vi "Get Category.vi"(8 "error in (no error)":errorcluster, 11 "WaveformAcq editor node in":refnum<class "WaveformAcq editor node.lvclass">) -> (0 "error out":errorcluster, 2 "Category":string, 3 "WaveformAcq editor node out":refnum<class "WaveformAcq editor node.lvclass">)   [LabVIEW 2017, in "WaveformAcq editor node.lvclass"]
uses:
  WaveformAcq editor node.lvclass
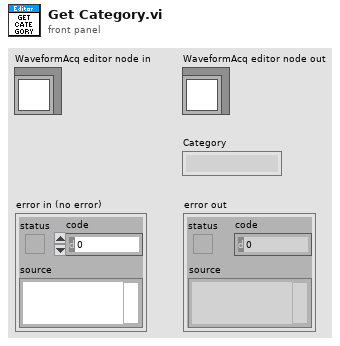
[diagram p1: front panel]
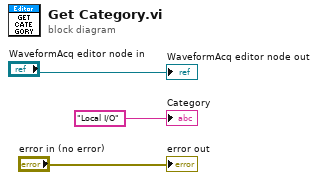
[diagram p0: block diagram]
diagram:
  "error out" <- "error in (no error)"
  "WaveformAcq editor node out" <- "WaveformAcq editor node in"
  "Category" <- "Local I/O" ("Category")
